vi "svfa_Tone Estimation Subroutine G(f).vi"   [LabVIEW 2017]
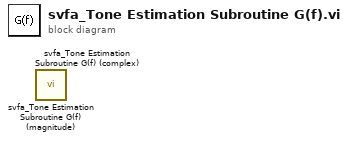
[diagram p0: block diagram]
diagram:
  n1 = call <vilib>:"svfa_Tone Estimation Subroutine G(f) (magnitude).vi"() -> ()  [unwired: 6 in, 2 out]
  n2 = call <vilib>:"svfa_Tone Estimation Subroutine G(f) (complex).vi"() -> ()  [unwired: 5 in, 3 out]
